vi "Actor Core.vi"(8 "error in":errorcluster, 11 "Connection Listener in":refnum<class "Connection Listener.lvclass">) -> (0 "error out":errorcluster, 3 "Actor out":refnum<class "Actor.lvclass">)   [LabVIEW 2017, in "Connection Listener.lvlib" / "Connection Listener.lvclass"]
doc: "(<B>Filename</B>: Actor Framework.lvlib:Actor.lvclass:Actor Core.vi)\n\nReceives messages to the actor, reacts to them, and initiates any error handling that may shut the actor down.\n\nDescendant classes may override this VI to append parallel tasks for the actor to complete while it handles messages. Overrides use the Call Parent Method node."
uses:
  Connection Listener.lvclass
  <vilib>/ActorFramework/Actor/Actor.lvclass
  Connection Listener.lvclass/Connection Listener.ctl
  Actor wHelper/Actor wHelper/Actor wHelper.lvclass
panel:
  out "Port":u16
  in  "String":string
  # "Headless Connection Listener"
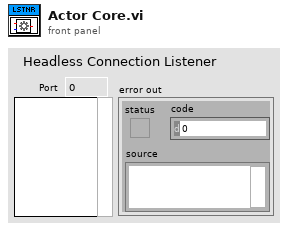
[diagram p1: front panel]
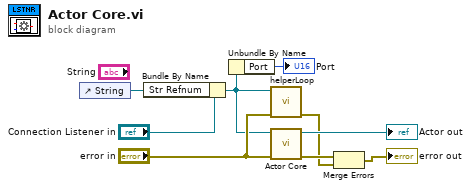
[diagram p0: block diagram]
diagram:
  n1 = control-ref of="String"() -> (w3:refnum<vi>)
  n2 = Bundle By Name(cluster="Connection Listener in", "Str Refnum"=w3) -> (w2:refnum<class "Connection Listener.lvclass">)
  n3 = Unbundle By Name(w2) -> ("Port"=→"Port":u16)
  n4 = call-dynamic "helperLoop.vi"("error in (no error)"="error in", "Connection Listener in"=w2) -> ("error out"=w4:errorcluster)  [unwired: 8 in, 1 out]
  n5 = call-parent "Actor Core.vi"("error in"="error in", "Actor in"=w2) -> ("error out"=w9:errorcluster, "Actor out"=→"Actor out":refnum<class "Actor.lvclass">)  [unwired: 8 in]
  n6 = Merge Errors(w9, w4) -> (→"error out":errorcluster)
